vi "DrawFormattedMulitLineString.vi"(0 "PictureIn":picture, 1 "FormattedMultiLineStringIn":string="123<B>ABCD</B>456\nAAA<B>BBB<I>CCC<U>DDD</U>EEE</I>FFF</B>GGG\n<I>QWERTY</I>\n<U>D<B>123</B>D</U>E", 2 "TextRectangle":T2={"x"=10.0, "y"=10.0, "width"=150.0, "height"=200.0} {"height" format="%.2f"; "width" format="%.2f"; "y" format="%.2f"; "x" format="%.2f"}, 3 "Justification":T1=enum."RIGHT", 4 "GAP":i32, 5 "Font":T3={"Font Name:"="Arial", "Size"=14, "Strikeout?"=FALSE, "Italic?"=FALSE, "Underline?"=FALSE, "Outline?"=FALSE, "Shadow?"=FALSE, "Bold?"=FALSE}, 6 "scaleY":dbl=2.0, 7 "Color":u32(colorbox), 8 "scaleX":dbl=2.0) -> (14 "PictureOut":picture)   [LabVIEW 2020, in "Graphics.lvclass"]
uses:
  <resource>/Framework/Providers/Open_GDS/UML/Graphics_class/Graphics.lvclass
  <resource>/Framework/Providers/Open_GDS/UML/General/Rectangle/Rectangle Rectangle2D.ctl
  <resource>/Framework/Providers/Open_GDS/UML/MultiLineString_class/JustificationType.ctl
  <resource>/Framework/Providers/Open_GDS/UML/MultiLineString_class/MultiLineString.lvclass
panel:
  # "Layout:\nRemove \\r\\n\nSplit in lines-array\nCalc width per char\nGet number of chars to use for line,\nif rest characters, add these to beggining of  lines-array.\nCalc Bound\nAdd \\r\\n where new lines breaks are"
  # "Drawing:\nRemove \\r, split line using \\n\nfor every line calc total length.\n\nFor each line\n  If left start\n  X=B.X+Gap\n  Right:\n  X=B.X+B.W-L.length-Gap\n  Center:\n  X=B.X+(B.W/2)-(L.length/2)\n  Draw Line\nEnd For"
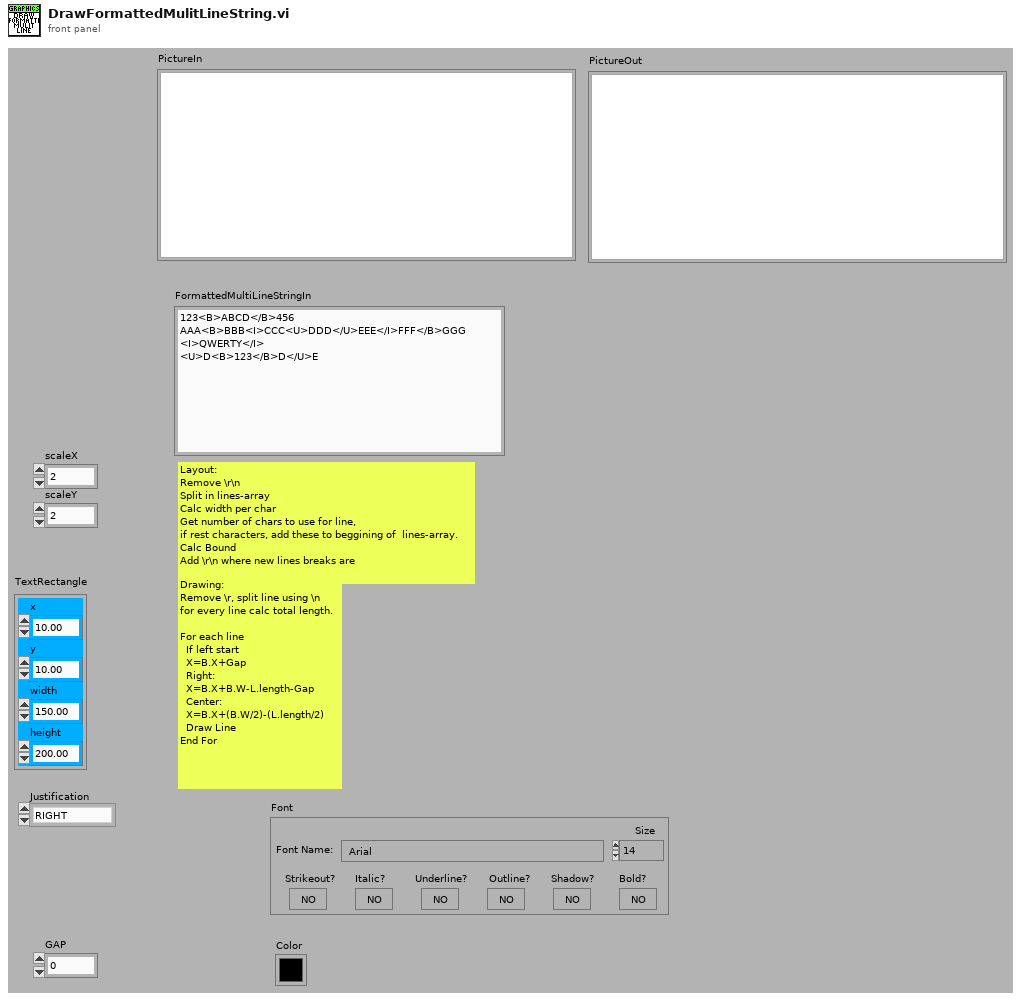
[diagram p1: front panel]
types:
  T1 = typedef "MultiLineString.lvclass/JustificationType.ctl" = enum16{"LEFT", "CENTER", "RIGHT"}
  T2 = typedef "Rectangle Rectangle2D.ctl" = cluster{"x":dbl, "y":dbl, "width":dbl, "height":dbl}
  T3 = cluster{"Font Name:":string, "Size":i16, "Strikeout?":bool, "Italic?":bool, "Underline?":bool, "Outline?":bool, "Shadow?":bool, "Bold?":bool}
  T4 = enum16{"User-specified Font", "Application Font", "System Font", "Dialog Font"}
  T5 = cluster{"Start":i32, "Stop":i32, "Font":cluster{"Font Name:":string, "Size":i16, "Strikeout?":bool, "Italic?":bool, "Underline?":bool, "Outline?":bool, "Shadow?":bool, "Bold?":bool}, "Color":u32}
  T6 = cluster{"Start":i32, "Stop":i32, "Font":cluster{"Font Name:":string, "Size":i16, "Strikeout?":bool, "Italic?":bool, "Underline?":bool, "Outline?":bool, "Shadow?":bool, "Bold?":bool}, "Color":u32}[]
  T7 = cluster{cluster{"Start":i32, "Stop":i32, "Font":cluster{"Font Name:":string, "Size":i16, "Strikeout?":bool, "Italic?":bool, "Underline?":bool, "Outline?":bool, "Shadow?":bool, "Bold?":bool}, "Color":u32}[]}
  T8 = cluster{"left":i16, "top":i16, "right":i16, "bottom":i16}
  T9 = cluster{"x":i16, "y":i16, "width":i16, "height":i16}
  T10 = cluster{"horizontal":enum16{"left", "center", "right"}, "vertical":enum16{"top", "center", "bottom"}}
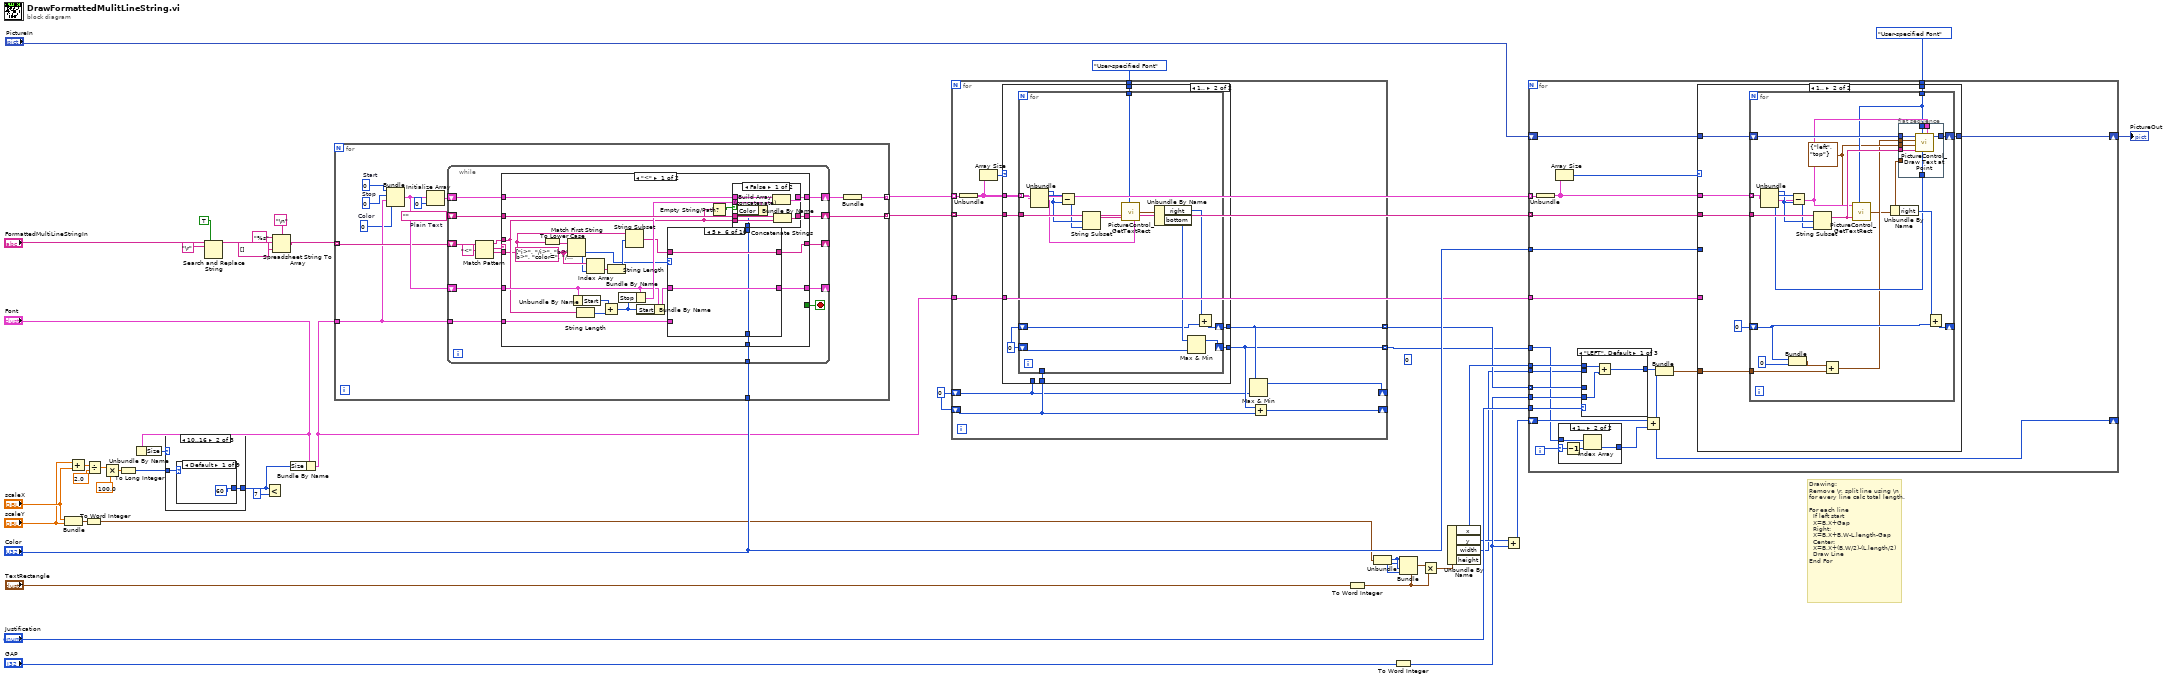
[diagram p0: block diagram]
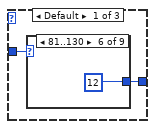
[diagram p2: hidden frame]
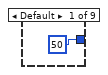
[diagram p3: hidden frame]
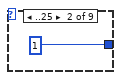
[diagram p4: hidden frame]
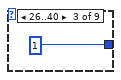
[diagram p5: hidden frame]
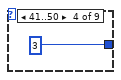
[diagram p6: hidden frame]
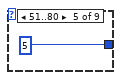
[diagram p7: hidden frame]
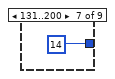
[diagram p8: hidden frame]
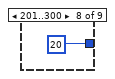
[diagram p9: hidden frame]
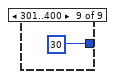
[diagram p10: hidden frame]
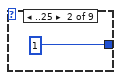
[diagram p11: hidden frame]
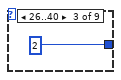
[diagram p12: hidden frame]
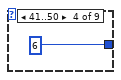
[diagram p13: hidden frame]
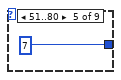
[diagram p14: hidden frame]
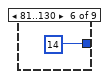
[diagram p15: hidden frame]
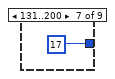
[diagram p16: hidden frame]
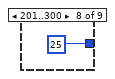
[diagram p17: hidden frame]
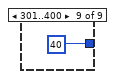
[diagram p18: hidden frame]
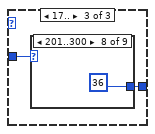
[diagram p19: hidden frame]
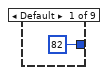
[diagram p20: hidden frame]
diagram:
  (unwired) 0 ("index")
  w41 = i16 0
  # "Drawing:\nRemove \\r, split line using \\n\nfor every line calc total length.\n\nFor each line\n  If left start\n  X=B.X+Gap\n  Right:\n  X=B.X+B.W-L.length-Gap\n  Center:\n  X=B.X+(B.W/2)-(L.length/2)\n  Draw Line\nEnd For"
  n1 = Bundle("scaleX"="scaleX", "scaleY"="scaleY") -> (w20:cluster{"scaleX":dbl, "scaleY":dbl})  [unwired: 1 out]
  n2 = Add(x="scaleY", y="scaleX") -> (x+y=w32:dbl)
  n3 = To Word Integer(number=w20) -> (16bit integer=w6:cluster{"scaleX":i16, "scaleY":i16})
  n4 = Divide(x=w32, y=2.0) -> (x/y=w30:dbl)
  n5 = Multiply(x=w30, y=100.0) -> (x*y=w28:dbl)
  n6 = To Long Integer(number=w28) -> (32bit integer=w27:i32)
  n7 = Unbundle By Name("Font") -> ("Size"=w22:i16)
  n8 = case shown="10..16" w22 {
    tunnel: [w48 w59 w69] -> w21
    tunnel: w27 -> [w47 w58 w70]
    frame Default {
      n9 = case shown="81..130" w47 {
        tunnel: [i16 50 ("Size 9") i16 1 ("Size") i16 1 ("Size 2") i16 3 ("Size 3") i16 5 ("Size 4") i16 12 ("Size 5") i16 14 ("Size 6") i16 20 ("Size 7") i16 30 ("Size 8")] -> w48
        frame Default {
        }
        frame ..25 {
        }
        frame 26..40 {
        }
        frame 41..50 {
        }
        frame 51..80 {
        }
        frame 81..130 {
        }
        frame 131..200 {
        }
        frame 201..300 {
        }
        frame 301..400 {
        }
      }
    }
    frame 10..16 {
      n10 = case shown="Default" w58 {
        tunnel: [i16 60 ("Size 9") i16 1 ("Size") i16 2 ("Size 2") i16 6 ("Size 3") i16 7 ("Size 4") i16 14 ("Size 5") i16 17 ("Size 6") i16 25 ("Size 7") i16 40 ("Size 8")] -> w59
        frame Default {
        }
        frame ..25 {
        }
        frame 26..40 {
        }
        frame 41..50 {
        }
        frame 51..80 {
        }
        frame 81..130 {
        }
        frame 131..200 {
        }
        frame 201..300 {
        }
        frame 301..400 {
        }
      }
    }
    frame 17.. {
      n11 = case shown="201..300" w70 {
        tunnel: [i16 82 ("Size") i16 2 ("Size") i16 5 ("Size") i16 7 ("Size") i16 12 ("Size") i16 18 ("Size") i16 26 ("Size") i16 36 ("Size") i16 55 ("Size")] -> w69
        frame Default {
        }
        frame ..25 {
        }
        frame 26..40 {
        }
        frame 41..50 {
        }
        frame 51..80 {
        }
        frame 81..130 {
        }
        frame 131..200 {
        }
        frame 201..300 {
        }
        frame 301..400 {
        }
      }
    }
  }
  n12 = Search and Replace String(replace all?=TRUE ("replace all? (F)"), input string="FormattedMultiLineStringIn", search string="\r" ("delimiter (Tab)")) -> (result string=w37:string)  [unwired: 5 in, 3 out]
  n13 = Less?(x=w21, y=i16 7) -> ()  [unwired: 1 out]
  n14 = Spreadsheet String To Array(delimiter (Tab)="\n", format string="%s", spreadsheet string=w37, array type (2D Dbl)=string[] []) -> (array=w44:string[])
  n15 = Bundle By Name(cluster="Font", "Size"=w21) -> (w9:T3)
  n16 = for {
    tunnel: w44 -> [w86] mode=indexing
    tunnel: w9 -> [w85]
    tunnel: [w84] -> w35 mode=indexing
    tunnel: [w82] -> w36 mode=indexing
    tunnel: "Color" -> [w80]
    w81 = u32 0  # Color
    w88 = ""  # Plain Text
    w91 = 0  # Stop
    w92 = 0  # Start
    n17 = Bundle("Start"=w92, "Stop"=w91, "Font"=w85, "Color"=w81) -> (w89:T5)  [unwired: 1 out]
    n18 = Initialize Array(w89, 0 ("dimension size")) -> (w90:T6)
    n19 = while {
      shift-right: [w99] -> w83
      shift-left: w90 -> [w102]
      shift-right: [w101] -> _
      shift-left: w86 -> [w107]
      shift-right: [w98] -> _
      shift-left: w89 -> [w100]
      tunnel: w85 -> [w96]
      shift-right: [w94] -> w84
      shift-left: w88 -> [w95]
      tunnel: w80 -> [w93]
      stop <- w97 stop-if-true
      n20 = Match Pattern(string=w107, regular expression="<") -> (before substring=w104:string, match substring=w105:string, after substring=w103:string)  [unwired: 2 out]
      n21 = case shown="\"<\"" w105 {
        tunnel: w104 -> [w118 w200]
        tunnel: w103 -> [w112 _]
        tunnel: w102 -> [w126 w206]
        tunnel: [w129 _] -> w101
        tunnel: w100 -> [w120 w201]
        tunnel: [w125 w205] -> w99
        tunnel: [w131 w204] -> w98
        tunnel: [_ TRUE] -> w97
        tunnel: w96 -> [w130 _]
        tunnel: w95 -> [w128 w207]
        tunnel: [w127 w208] -> w94
        tunnel: w93 -> [w108 w198]
        frame "<" {
          w114 = string[] ["i>", "/i>", "b>", "/b>", "color=", "/color>", "u>", "/u>", "size=", "/size>"] ("string array")
          n22 = To Lower Case(string=w112) -> (all lower case string=w113:string)
          n23 = Match First String(2:w114, 3:w113) -> (0:w110:i32)  [unwired: 1 out]
          n24 = Unbundle By Name(w120) -> ("Start"=w123:i32)
          n25 = String Length(string=w118) -> (length=w124:i32)
          n26 = Index Array(array=w114, index=w110) -> (element=w115:string)
          n27 = Add(x=w123, y=w124) -> (x+y=w121:i32)
          n28 = String Length(string=w115) -> (length=w116:i32)
          n29 = Bundle By Name(cluster=w120, "Stop"=w121) -> (w122:T5)
          n30 = String Subset(string=w112, offset (0)=w116) -> (substring=w111:string)  [unwired: 1 in]
          n31 = Bundle By Name(cluster=w120, "Start"=w121) -> (w119:T5)
          n32 = case shown="5" w110 {
            tunnel: w119 -> [w144 w151 w155 w162 w164 w171 w175 w182 w190 w196]
            tunnel: [w146 w152 w157 w163 w164 w171 w177 w183 w191 w197] -> w131
            tunnel: w130 -> [_ w150 _ w161 _ _ _ w181 _ w194]
            tunnel: w111 -> [w143 w148 w154 w159 w169 w172 w174 w179 w189 w195]
            tunnel: [w143 w148 w154 w159 w166 w172 w174 w179 w185 w195] -> w129
            tunnel: [w142 w147 w153 w158 w165 w170 w173 w178 w184 w192] -> w109
            tunnel: w108 -> [w142 w147 w153 w158 _ w170 w173 w178 w184 w192]
            frame 0, Default {
              n33 = Bundle By Name(cluster=w144, "Font.Italic?"=TRUE ("Default Properties.Italic?")) -> (w146:T5)
            }
            frame 1 {
              n34 = Unbundle By Name(w150) -> ("Italic?"=w149:bool)
              n35 = Bundle By Name(cluster=w151, "Font.Italic?"=w149) -> (w152:T5)
            }
            frame 2 {
              n36 = Bundle By Name(cluster=w155, "Font.Bold?"=TRUE ("Default Properties.Italic?")) -> (w157:T5)
            }
            frame 3 {
              n37 = Unbundle By Name(w161) -> ("Bold?"=w160:bool)
              n38 = Bundle By Name(cluster=w162, "Font.Bold?"=w160) -> (w163:T5)
            }
            frame 4 {
              n39 = Scan From String(format string="%x>", input string=w169, default 1=u32 0 ("default value 1")) -> (remaining string=w166:string, output 1=w165:u32)  [unwired: 2 in, 2 out]
            }
            frame 5 {
            }
            frame 6 {
              n40 = Bundle By Name(cluster=w175, "Font.Underline?"=TRUE ("Default Properties.Italic?")) -> (w177:T5)
            }
            frame 7 {
              n41 = Unbundle By Name(w181) -> ("Underline?"=w180:bool)
              n42 = Bundle By Name(cluster=w182, "Font.Underline?"=w180) -> (w183:T5)
            }
            frame 8 {
              n43 = Scan From String(format string="%d>", input string=w189, default 1=i16 0 ("default value 1")) -> (remaining string=w185:string, output 1=w187:i16)  [unwired: 2 in, 2 out]
              n44 = Bundle By Name(cluster=w190, "Font.Size"=w187) -> (w191:T5)
            }
            frame 9 {
              n45 = Unbundle By Name(w194) -> ("Size"=w193:i16)
              n46 = Bundle By Name(cluster=w196, "Font.Size"=w193) -> (w197:T5)
            }
          }
          n47 = Empty String/Path?(string/path=w118) -> (empty?=w117:bool)
          n48 = case shown="False" w117 {
            tunnel: w128 -> [w139 w140]
            tunnel: [w138 w140] -> w127
            tunnel: w126 -> [w137 w141]
            tunnel: [w136 w141] -> w125
            tunnel: w122 -> [w134 _]
            tunnel: w118 -> [w135 _]
            tunnel: w109 -> [w132 _]
            frame False {
              n49 = Bundle By Name(cluster=w134, "Color"=w132) -> (w133:T5)
              n50 = Build Array (concatenate)(w137, w133) -> (w136:T6)
              n51 = Concatenate Strings(w139, w135) -> (w138:string)
            }
            frame True {
            }
          }
        }
        frame "", Default {
          n52 = Unbundle By Name(w201) -> ("Start"=w202:i32)
          n53 = String Length(string=w200) -> (length=w203:i32)
          n54 = Add(x=w202, y=w203) -> (x+y=w199:i32)
          n55 = Concatenate Strings(w207, w200) -> (w208:string)
          n56 = Bundle By Name(cluster=w201, "Stop"=w199, "Color"=w198) -> (w204:T5)
          n57 = Build Array (concatenate)(w206, w204) -> (w205:T6)
        }
      }
    }
    n58 = Bundle(w83) -> (w82:T7)  [unwired: 1 in]
  }
  n59 = for {
    tunnel: w36 -> [w221] mode=indexing
    tunnel: w35 -> [w220] mode=indexing
    tunnel: T4."User-specified Font" ("desired font(Application)") -> [w219]
    shift-right: [w218] -> _
    shift-left: w41 -> [w211]
    shift-right: [w217] -> _
    shift-left: w41 -> [w210]
    tunnel: [w216] -> w16 mode=indexing
    tunnel: [w215] -> w11 mode=indexing
    tunnel: w9 -> [w212]
    n60 = Unbundle(w221) -> (w214:T6)
    n61 = Array Size(array=w214) -> (size(s)=w213:i32)
    n62 = case shown="1.." w213 {
      tunnel: w220 -> [w223 w234]
      tunnel: w219 -> [w224 w233]
      tunnel: [w225 w231] -> w216
      tunnel: [w226 w230] -> w215
      tunnel: w214 -> [_ w229]
      tunnel: w212 -> [w222 _]
      tunnel: w211 -> [_ w228]
      tunnel: w210 -> [_ _]
      frame 0, Default {
        n63 = call <resource>:"PictureControl_GetTextRect.vi"("desired font(Application)"=w224, "text"=w223, "[user-specified font]"=w222) -> ("rect"=w227:T8)  [unwired: 6 in]
        n64 = Unbundle By Name(w227) -> ("right"=w225:i16, "bottom"=w226:i16)
      }
      frame 1.. {
        w232 = i16 0
        n65 = for {
          tunnel: w234 -> [w248]
          tunnel: w229 -> [w249] mode=indexing
          tunnel: w233 -> [w236]
          shift-right: [w239] -> w231
          shift-left: w232 -> [w237]
          shift-right: [w241] -> w230
          shift-left: w232 -> [w242]
          tunnel: w228 -> [_]
          n66 = Unbundle(w249) -> ("Start"=w246:i32, "Stop"=w247:i32, "Font"=w235:T3)  [unwired: 1 out]
          n67 = Subtract(x=w247, y=w246) -> (x-y=w245:i32)
          n68 = String Subset(string=w248, offset (0)=w246, length (rest)=w245) -> (substring=w238:string)
          n69 = call <resource>:"PictureControl_GetTextRect.vi"("desired font(Application)"=w236, "text"=w238, "[user-specified font]"=w235) -> ("rect"=w244:T8)  [unwired: 6 in]
          n70 = Unbundle By Name(w244) -> ("right"=w240:i16, "bottom"=w243:i16)
          n71 = Max & Min(x=w243, y=w242) -> (max(x,y)=w241:i16)  [unwired: 1 out]
          n72 = Add(x=w240, y=w237) -> (x+y=w239:i16)
        }
      }
    }
    n73 = Max & Min(x=w216, y=w210) -> (max(x,y)=w217:i16)  [unwired: 1 out]
    n74 = Add(x=w215, y=w211) -> (x+y=w218:i16)
  }
  n75 = To Word Integer(number="TextRectangle") -> (16bit integer=w3:T9)
  n76 = Unbundle(w6) -> ("scaleX"=w5:i16, "scaleY"=w4:i16)
  n77 = To Word Integer(number="GAP") -> (16bit integer=w15:i16)
  n78 = Bundle(cluster=w3, "x"=w5, "y"=w4, "width"=w5, "height"=w4) -> (w2:T9)
  n79 = Multiply(x=w2, y=w3) -> (x*y=w7:T9)
  n80 = Unbundle By Name(w7) -> ("x"=w19:i16, "y"=w14:i16, "width"=w10:i16)  [unwired: 1 out]
  n81 = Add(x=w14, y=w15) -> (x+y=w13:i16)
  n82 = for {
    tunnel: w36 -> [w270] mode=indexing
    tunnel: w35 -> [w269] mode=indexing
    tunnel: w9 -> [w266]
    shift-right: [w264] -> w34
    shift-left: "PictureIn" -> [w265]
    tunnel: "Color" -> [w263]
    tunnel: w19 -> [w257]
    tunnel: "Justification" -> [w258]
    tunnel: w15 -> [w260]
    tunnel: w16 -> [w259] mode=indexing
    tunnel: w11 -> [w253]
    shift-right: [w255] -> _
    shift-left: w13 -> [w261]
    tunnel: T4."User-specified Font" ("desired font(Application)") -> [w254]
    tunnel: w10 -> [w250]
    i -> [w251]
    n83 = Unbundle(w270) -> (w268:T6)
    n84 = Array Size(array=w268) -> (size(s)=w267:i32)
    n85 = case shown="1.." w251 {
      selector: w251 -> [_ w271]
      tunnel: w253 -> [_ w274]
      tunnel: [_ w272] -> w252
      frame 0, Default {
      }
      frame 1.. {
        n86 = Decrement(x=w271) -> (x-1=w273:i32)
        n87 = Index Array(array=w274, index=w273) -> (element=w272:i16)
      }
    }
    n88 = case shown="\"LEFT\", Default" w258 {
      tunnel: w259 -> [_ w280 w287]
      tunnel: w257 -> [w277 w278 w292]
      tunnel: w260 -> [w276 w284 _]
      tunnel: [w275 w283 w291] -> w262
      tunnel: w250 -> [_ w279 w290]
      frame "LEFT", Default {
        n89 = Add(x=w277, y=w276) -> (x+y=w275:i16)
      }
      frame "RIGHT" {
        n90 = Add(x=w278, y=w279) -> (x+y=w282:i16)
        n91 = Subtract(x=w282, y=w280) -> (x-y=w281:i16)
        n92 = Subtract(x=w281, y=w284) -> (x-y=w283:i16)
      }
      frame "CENTER" {
        w286 = 2.0 ("y")
        n93 = Divide(x=w290, y=w286) -> (x/y=w293:dbl)
        n94 = Divide(x=w287, y=w286) -> (x/y=w285:dbl)
        n95 = Add(x=w292, y=w293) -> (x+y=w289:dbl)
        n96 = Subtract(x=w289, y=w285) -> (x-y=w288:dbl)
        n97 = To Word Integer(number=w288) -> (16bit integer=w291:i16)
      }
    }
    n98 = Add(x=w261, y=w252) -> (x+y=w255:i16)
    n99 = Bundle(w262, w255) -> (w256:cluster{i16, i16})  [unwired: 1 in]
    n100 = case shown="1.." w267 {
      tunnel: w269 -> [w299 w308]
      tunnel: w268 -> [_ w306]
      tunnel: w266 -> [w296 _]
      tunnel: w265 -> [w301 w305]
      tunnel: [w300 w304] -> w264
      tunnel: w263 -> [w297 _]
      tunnel: w256 -> [w294 w302]
      tunnel: w254 -> [w295 w303]
      frame 0, Default {
        n101 = call <resource>:"PictureControl_Draw Text at Point.vi"("[user-specified font]"=w296, "text color(black)"=w297, "desired font(Application)"=w295, "text"=w299, "alignment(left, top)"=T10 {"horizontal"=enum."left", "vertical"=enum."top"}, "origin"=w294, "picture"=w301) -> ("new picture"=w300:picture)  [unwired: 3 in, 1 out]
      }
      frame 1.. {
        n102 = for {
          tunnel: w308 -> [w327]
          tunnel: w306 -> [w328] mode=indexing
          shift-right: [w322] -> _
          shift-left: i16 0 -> [w318]
          shift-right: [w320] -> w304
          shift-left: w305 -> [w321]
          tunnel: w302 -> [w315]
          tunnel: w303 -> [w312]
          w311 = T10 {"horizontal"=enum."left", "vertical"=enum."top"} ("alignment(left, top)")
          n103 = Unbundle(w328) -> ("Start"=w325:i32, "Stop"=w326:i32, "Font"=w316:T3, "Color"=w317:u32)
          n104 = Bundle(w318, i16 0) -> (w314:cluster{i16, i16})  [unwired: 1 in]
          n105 = Subtract(x=w326, y=w325) -> (x-y=w324:i32)
          n106 = String Subset(string=w327, offset (0)=w325, length (rest)=w324) -> (substring=w319:string)
          n107 = Add(x=w314, y=w315) -> (x+y=w310:cluster{i16, i16})
          n108 = call <resource>:"PictureControl_GetTextRect.vi"("alignment(left, top)"=w311, "desired font(Application)"=w312, "text"=w319, "[user-specified font]"=w316) -> ("rect"=w309:T8)  [unwired: 5 in]
          n109 = Unbundle By Name(w309) -> ("right"=w323:i16)
          n110 = flat-sequence {
            tunnel: w321 -> [w336]
            tunnel: [w335] -> w320
            tunnel: w319 -> [w334]
            tunnel: w317 -> [w333]
            tunnel: w316 -> [w332]
            tunnel: w312 -> [w331]
            tunnel: w311 -> [w330]
            tunnel: w310 -> [w329]
            tunnel: w309 -> [_]
            frame #0 {
              n111 = call <resource>:"PictureControl_Draw Text at Point.vi"("[user-specified font]"=w332, "text color(black)"=w333, "desired font(Application)"=w331, "text"=w334, "alignment(left, top)"=w330, "origin"=w329, "picture"=w336) -> ("new picture"=w335:picture)  [unwired: 3 in, 1 out]
            }
          }
          n112 = Add(x=w323, y=w318) -> (x+y=w322:i16)
        }
      }
    }
  }
  "PictureOut" <- w34
